vi "Change Panel State.vi"(8 "error in (no error)":errorcluster, 10 "Open/Close":bool, 11 "UserInterface in":refnum<class "UserInterface.lvclass">) -> (0 "error out":errorcluster)   [LabVIEW 2016, in "UserInterface.lvlib" / "UserInterface.lvclass"]
uses:
  UserInterface.lvclass
  UserInterface.lvclass/UserInterface.ctl
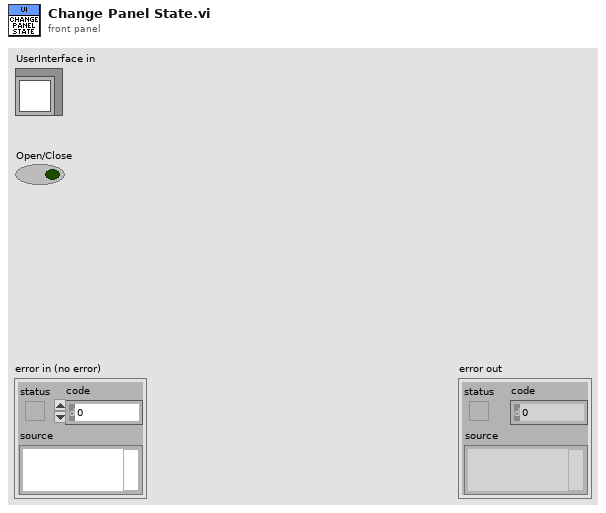
[diagram p1: front panel]
types:
  T1 = enum32{"Invalid", "Standard", "Closed", "Hidden", "Minimized", "Maximized"}
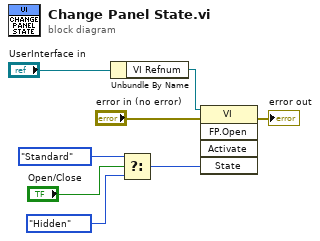
[diagram p0: block diagram]
diagram:
  n1 = Unbundle By Name("UserInterface in") -> ("VI Refnum"=w7:refnum<vi>)
  n2 = Select(t=T1."Standard" ("State"), s="Open/Close", f=T1."Hidden" ("State")) -> (s? t:f=w3:T1)
  n3 = invoke class="VI" method="FP.Open"(reference=w7, error in="error in (no error)", "State"=w3) -> (error out=→"error out":errorcluster)  [unwired: 2 in, 4 out]
